vi "R2D2.VI"(8 "error in (no error)":errorcluster, 10 "Min Frequency (Hz)":i32=200, 11 "Number of Notes":i32=8) -> (0 "error out":errorcluster)   [LabVIEW 2020]
panel:
  in  "Max Frequency (Hz)":i32=2000
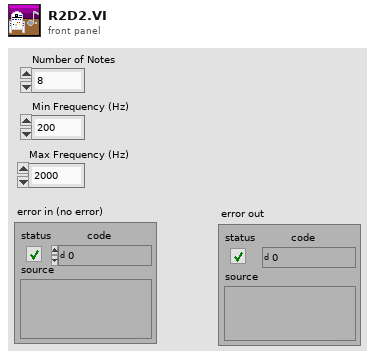
[diagram p1: front panel]
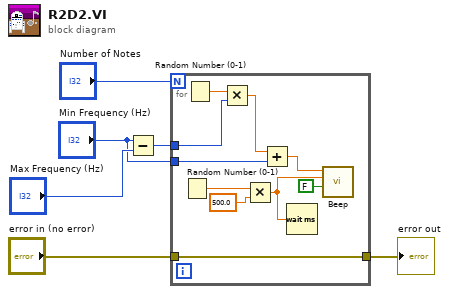
[diagram p0: block diagram]
diagram:
  n1 = Subtract(x="Min Frequency (Hz)", y="Max Frequency (Hz)") -> (x-y=w4:i32)
  n2 = for {
    N: "Number of Notes" -> [_]
    tunnel: w4 -> [w12]
    tunnel: "Min Frequency (Hz)" -> [w10]
    tunnel: [w8] -> w2
    tunnel: "error in (no error)" -> [w8]
    n3 = Random Number (0-1)() -> (number: 0 to 1=w14:dbl)
    n4 = Random Number (0-1)() -> (number: 0 to 1=w13:dbl)
    n5 = Multiply(x=w13, y=w12) -> (x*y=w11:dbl)
    n6 = Multiply(x=w14, y=500.0) -> (x*y=w7:dbl)
    n7 = Add(x=w11, y=w10) -> (x+y=w9:dbl)
    n8 = Wait (ms)(milliseconds to wait=w7) -> ()  [unwired: 1 out]
    n9 = call <vilib>:"Beep.vi"("use system alert? (T)"=FALSE, "duration (msec)"=w7, "frequency (Hz)"=w9) -> ()  [unwired: 9 in]
  }
  "error out" <- w2
